vi "Lab2_Exercise3a_Li_Lim.vi"() -> ()   [LabVIEW 2016]
panel:
  out "String":string
  in  "Write ur text here":string
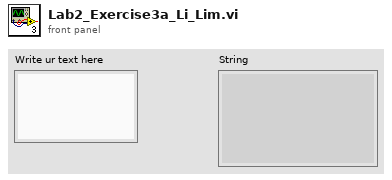
[diagram p1: front panel]
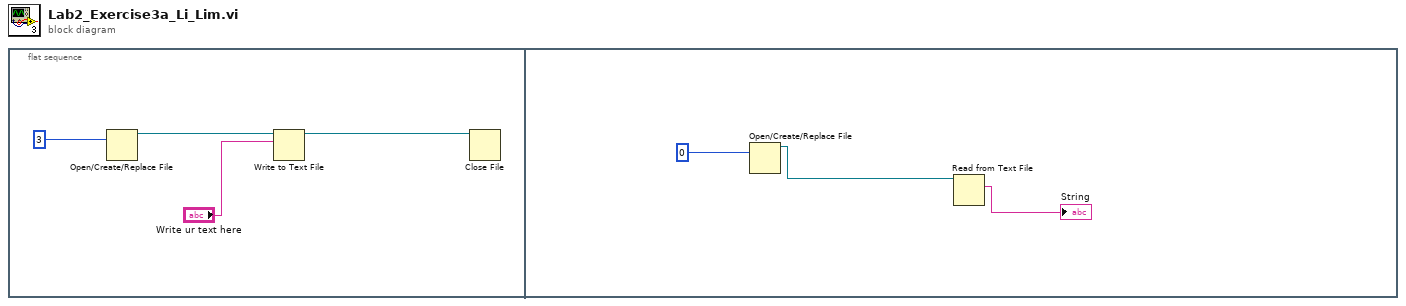
[diagram p0: block diagram]
diagram:
  n1 = flat-sequence {
    frame #0 {
      n2 = Open/Create/Replace File(operation (0:open)=3) -> (refnum out=w3:refnum<file>)  [unwired: 5 in, 2 out]
      n3 = Write to Text File(file (use dialog)=w3, text="Write ur text here") -> (refnum out=w2:refnum<file>)  [unwired: 2 in, 2 out]
      n4 = Close File(refnum=w2) -> ()  [unwired: 1 in, 2 out]
    }
    frame #1 {
      n5 = Open/Create/Replace File(operation (0:open)=0) -> (refnum out=w5:refnum<file>)  [unwired: 5 in, 2 out]
      n6 = Read from Text File(file (use dialog)=w5) -> (text=→"String":string)  [unwired: 3 in, 3 out]
    }
  }
